vi "2D Animate Rotating Wheel.vi"(6 "degree (T)":bool, 8 "Angle":dbl format="%.2f") -> (3 "new picture":picture)   [LabVIEW 2017]
uses:
  <vilib>/picture/picture.llb/imagedata.ctl
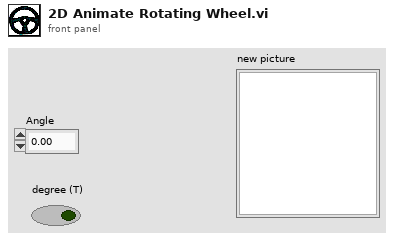
[diagram p1: front panel]
types:
  T1 = typedef "imagedata.ctl" = cluster{"image type":i32, "image depth":i32, "image":u8[], "mask":u8[], "colors":u32[], "Rectangle":cluster{"left":i16, "top":i16, "right":i16, "bottom":i16}}
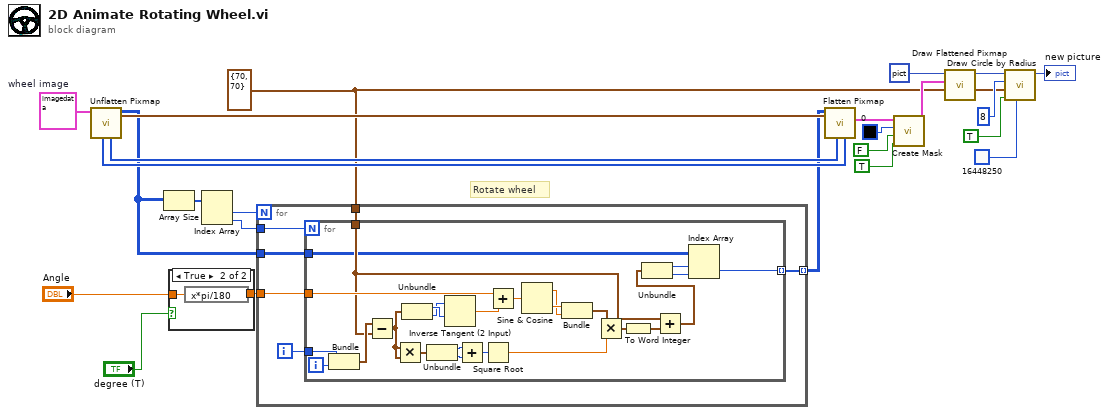
[diagram p0: block diagram]
diagram:
  w21 = T1 {"image type"=0, "image depth"=24, "image"=array[58800 elements], "mask"=[], "colors"=[], "Rectangle"={"left"=0, "top"=0, "right"=140, "bottom"=140}}  # wheel image
  w4 = cluster{"x":i16, "y":i16} {"x"=70, "y"=70} ("Center 2")
  # "Rotate wheel"
  n1 = call <vilib>:"Unflatten Pixmap.vi"("image data"=w21) -> ("24-bit pixmap"=w3:u32[][], "colors"=w19:u32[], "top left"=w20:cluster{"x":i16, "y":i16}, "mask"=w11:u8[])  [unwired: 7 out]
  n2 = Array Size(array=w3) -> (size(s)=w24:i32[])
  n3 = case shown="True" "degree (T)" {
    tunnel: [w25 w27] -> w7
    tunnel: "Angle" -> [w25 w26]
    frame False {
    }
    frame True {
      n4 = expression code="x*pi/180"(w26) -> (w27:dbl)
    }
  }
  n5 = Index Array(array=w24) -> (element #1=w22:i32, element #2=w23:i32)  [unwired: 2 in]
  n6 = for {
    N: w22 -> [_]
    tunnel: w23 -> [w33]
    tunnel: w7 -> [w32]
    tunnel: w4 -> [w31]
    tunnel: w3 -> [w29]
    tunnel: [w28] -> w2 mode=indexing
    i -> [w30]
    n7 = for {
      N: w33 -> [_]
      tunnel: w30 -> [w58]
      tunnel: w32 -> [w48]
      tunnel: w31 -> [w37]
      tunnel: w29 -> [w35]
      tunnel: [w34] -> w28 mode=indexing
      i -> [w36]
      n8 = Bundle(w58, w36) -> (w57:cluster{i32, i32})  [unwired: 1 out]
      n9 = Subtract(x=w57, y=w37) -> (x-y=w52:cluster{i32, i32})
      n10 = Multiply(x=w52, y=w52) -> (x*y=w56:cluster{i32, i32})
      n11 = Unbundle(w52) -> (w51:i32, w50:i32)
      n12 = Unbundle(w56) -> (w55:i32, w54:i32)
      n13 = Inverse Tangent (2 Input)(1:w51, 2:w50) -> (0:w49:dbl)
      n14 = Add(x=w55, y=w54) -> (x+y=w53:i32)
      n15 = Square Root(x=w53) -> (sqrt(x)=w43:dbl)
      n16 = Add(x=w48, y=w49) -> (x+y=w47:dbl)
      n17 = Sine & Cosine(0:w47) -> (1:w45:dbl, 2:w46:dbl)
      n18 = Bundle(w46, w45) -> (w44:cluster{dbl, dbl})  [unwired: 1 out]
      n19 = Multiply(x=w44, y=w43) -> (x*y=w42:cluster{dbl, dbl})
      n20 = To Word Integer(number=w42) -> (16bit integer=w41:cluster{i16, i16})
      n21 = Add(x=w37, y=w41) -> (x+y=w38:cluster{i16, i16})
      n22 = Unbundle(w38) -> (w40:i16, w39:i16)
      n23 = Index Array(array=w35, index (row)=w40, index (col)=w39) -> (element=w34:u32)
    }
  }
  n24 = call <vilib>:"Flatten Pixmap.vi"("mask"=w11, "colors"=w19, "top left"=w20, "24-bit pixmap"=w2) -> ("image data"=w13:T1)  [unwired: 3 in, 4 out]
  n25 = call <vilib>:"Create Mask.vi"("Combine Masks? (F)"=TRUE, "1-Bit Mask Value (T)"=FALSE, "Mask Color (Black)"=u32 0, "image data"=w13) -> ("image data"=w12:T1)  [unwired: 7 out]
  n26 = call <vilib>:"Draw Flattened Pixmap.vi"("image data"=w12, "picture"=picture data[5B]) -> ("new picture"=w18:picture)  [unwired: 7 out]
  n27 = call <vilib>:"Draw Circle by Radius.vi"("color(black)"=u32 16448250, "fill?(F)"=TRUE, "pixel center"=w4, "radius"=i16 8, "picture"=w18) -> ("new picture"=→"new picture":picture)  [unwired: 3 in, 3 out]
